vi "Check Right Click.vi"(9 "Ctrl":bool, 11 "Button":u16) -> (3 "Right Click?":bool)   [LabVIEW 2017, in "3D Plot.lvclass"]
uses:
  <vilib>/Math Plots/3D Math Plots/3D Plot/3D Plot/3D Plot.lvclass
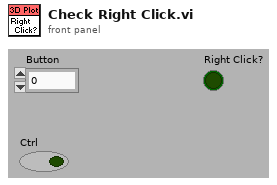
[diagram p1: front panel]
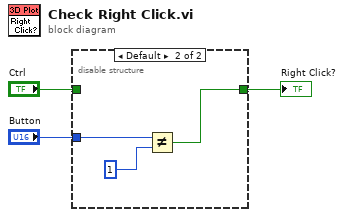
[diagram p0: block diagram]
diagram:
  n1 = disable-structure shown="Default" {
    disable-tunnel: "Button" -> [_ w7]
    disable-tunnel: [w4 w5] -> w2
    disable-tunnel: "Ctrl" -> [w4 _]
    frame condition #0 {
    }
    frame condition #1 (active) {
      n2 = Not Equal?(x=w7, y=u16 1) -> (x != y?=w5:bool)
    }
  }
  "Right Click?" <- w2
